vi "DestroyModuleBroadcasts.vi"(8 "error in (no error)":errorcluster, 11 "JQMHModule in":refnum<class "RQMHModule.lvclass">) -> (0 "error out":errorcluster, 3 "JQMHModule out":refnum<class "RQMHModule.lvclass">)   [LabVIEW 2024, in "RQMHModule.lvclass"]
uses:
  RQMHModule.lvclass
  RQMHModule.lvclass/RQMHModule.ctl
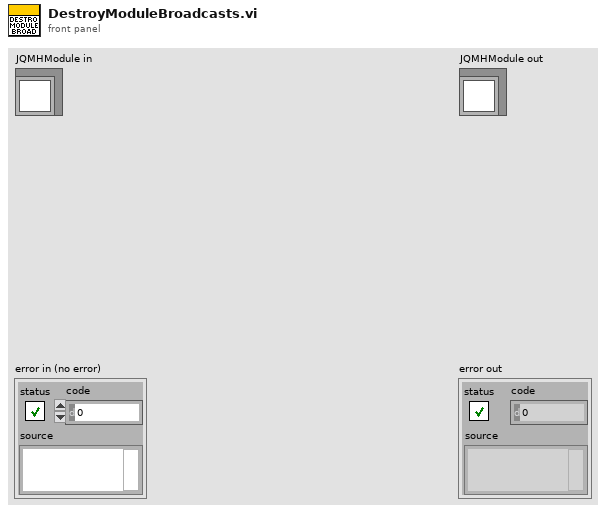
[diagram p1: front panel]
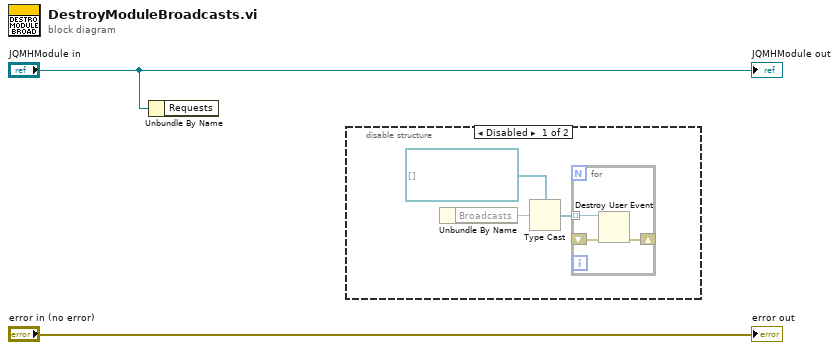
[diagram p0: block diagram]
diagram:
  n1 = Unbundle By Name("JQMHModule in") -> ()  [unwired: 1 out]
  n2 = disable-structure shown="Disabled" {
    frame Disabled {
      n3 = Unbundle By Name() -> (w4:refnum<class "TesterModule.lvclass">, "Broadcasts"=w6)
      n4 = Type Cast(type=refnum<user-event>[] [] ("NewControl5"), x=w6) -> (*(type *) &x=w5:refnum<user-event>[])
      n5 = for {
        tunnel: w5 -> [w10] mode=indexing
        shift-right: [w8] -> _
        shift-left: [w9] -> w3
        n6 = Destroy User Event(user event=w10, error in=w9) -> (error out=w8:errorcluster)
      }
    }
    frame Enabled {
    }
  }
  "error out" <- "error in (no error)"
  "JQMHModule out" <- "JQMHModule in"
